vi "Get Number New Images.vi"(10 "last":i32, 11 "first":i32) -> (1 "function return":u32, 2 "last out":i32, 3 "first out":i32)   [LabVIEW 2018, in "Copy of Andor SDK.lvlib"]
doc: "EXPNETTYPE unsigned int WINAPI GetNumberNewImages(long * first, long * last);"
uses:
  Copy of Andor SDK.lvlib
  <userlib>/Andor SDK/ATMCD32D.dll
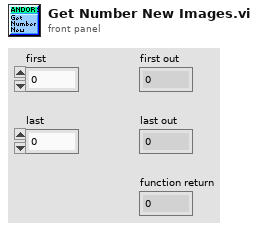
[diagram p1: front panel]
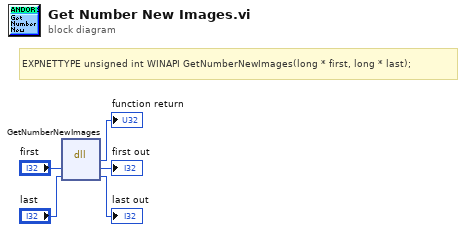
[diagram p0: block diagram]
diagram:
  # "EXPNETTYPE unsigned int WINAPI GetNumberNewImages(long * first, long * last);"
  n1 = dll-call lib="C:/Program Files (x86)/National Instruments/LabVIEW 2018/user.lib/Andor SDK/ATMCD32D.*" fn="GetNumberNewImages"("first"="first", "last"="last") -> (→"function return":u32, "first"=→"first out":i32, "last"=→"last out":i32)  [unwired: 3 in, 2 out]
